vi "Network_Ping.vi"(4 "dontFragment (F)":bool, 6 "Bytes number (32)":u16=32, 8 "error in (no error)":errorcluster, 9 "Tentatives (4)":u16(ring)=4 items=["1"=1, "2"=2, "3"=3, "4"=4], 10 "TimeOut (100ms)":i32=100, 11 "Address":string="localhost") -> (0 "error out":errorcluster, 1 "Success":bool, 2 "Status":i32(ring) items=["Success"=0, "DestinationNetworkUnreachable"=11002, "DestinationHostUnreachable"=11003, "DestinationProhibited, DestinationProtocolUnreachable"=11004, "DestinationPortUnreachable"=11005, "NoResources"=11006, "BadOption"=11007, "HardwareError"=11008, "PacketTooBig"=11009, "TimedOut"=11010, "BadRoute"=11012, "TtlExpired"=11013, "TtlReassemblyTimeExceeded"=11014, "ParameterProblem"=11015, "SourceQuench"=11016, "BadDestination"=11018, "DestinationUnreachable"=11040, "TimeExceeded"=11041, "BadHeader"=11042, "UnrecognizedNextHeader"=11043, "IcmpError"=11044, "DestinationScopeMismatch"=11045, "Unknown"=-1])   [LabVIEW 2021]
doc: "This VI sends n ping to an address.\n\n.NET Technology, works only for Windows."
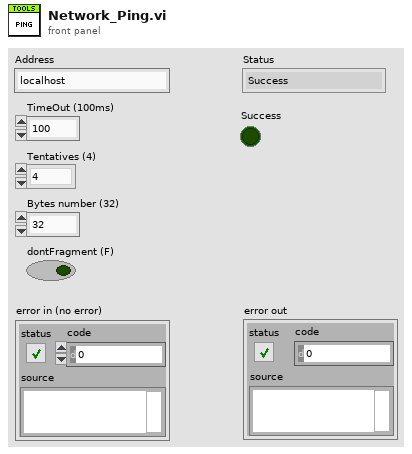
[diagram p1: front panel]
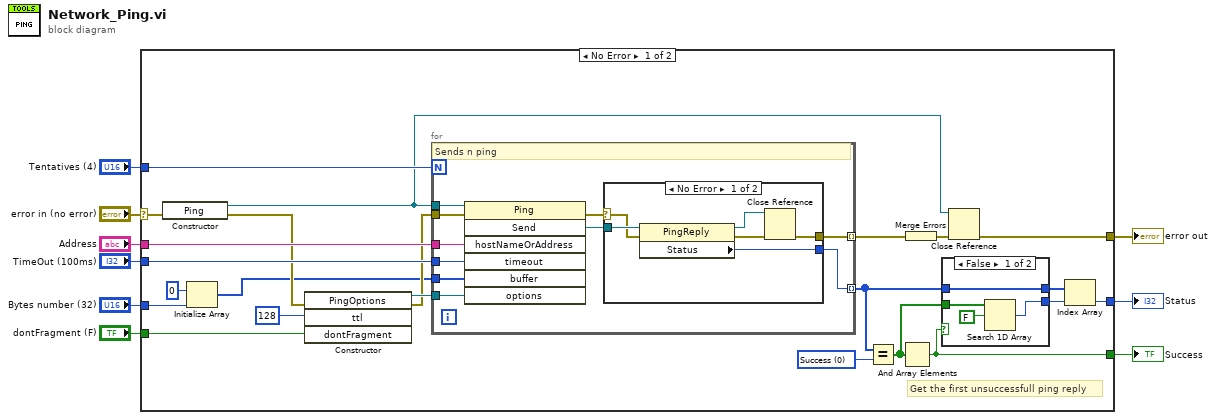
[diagram p0: block diagram]
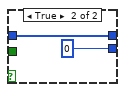
[diagram p2: hidden frame]
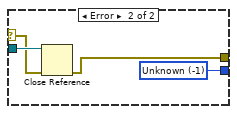
[diagram p3: hidden frame]
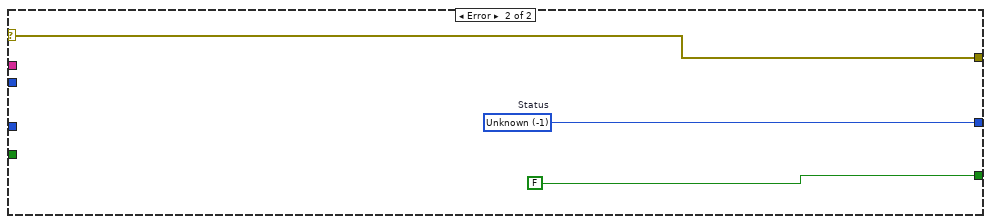
[diagram p4: hidden frame]
diagram:
  n1 = case shown="No Error" "error in (no error)" {
    selector: "error in (no error)" -> [w21 w61]
    tunnel: "Address" -> [w32 _]
    tunnel: "TimeOut (100ms)" -> [w31 _]
    tunnel: "Tentatives (4)" -> [w30 _]
    tunnel: [w26 w61] -> w6
    tunnel: [w24 FALSE] -> w5
    tunnel: [w22 w60] -> w4
    tunnel: "Bytes number (32)" -> [w14 _]
    tunnel: "dontFragment (F)" -> [w10 _]
    frame No Error {
      w19 = 0 items=["Success"=0, "DestinationNetworkUnreachable"=11002, "DestinationHostUnreachable"=11003, "DestinationProhibited, DestinationProtocolUnreachable"=11004, "DestinationPortUnreachable"=11005, "NoResources"=11006, "BadOption"=11007, "HardwareError"=11008, "PacketTooBig"=11009, "TimedOut"=11010, "BadRoute"=11012, "TtlExpired"=11013, "TtlReassemblyTimeExceeded"=11014, "ParameterProblem"=11015, "SourceQuench"=11016, "BadDestination"=11018, "DestinationUnreachable"=11040, "TimeExceeded"=11041, "BadHeader"=11042, "UnrecognizedNextHeader"=11043, "IcmpError"=11044, "DestinationScopeMismatch"=11045, "Unknown"=-1] ("Status")
      # "Get the first unsuccessfull ping reply"
      n2 = constructor class="Ping"(error in=w21) -> (reference out=w28:refnum<k24>, error out=w15:errorcluster)  [unwired: 2 in, 1 out]
      n3 = Initialize Array(u8 0, w14) -> (w12:u8[])
      n4 = constructor class="PingOptions"(error in=w15, "ttl"=128, "dontFragment"=w10) -> (reference out=w17:refnum<k24>, error out=w16:errorcluster)  [unwired: 2 in, 3 out]
      n5 = for {
        N: w30 -> [_]
        tunnel: w28 -> [w48]
        tunnel: w32 -> [w46]
        tunnel: w31 -> [w45]
        tunnel: w16 -> [w47]
        tunnel: [w42] -> w29 mode=indexing
        tunnel: [w41] -> w20 mode=indexing
        tunnel: w12 -> [w40]
        tunnel: w17 -> [w39]
        # "Sends n ping"
        n6 = invoke class="Ping" method="Send"(reference=w48, error in=w47, "hostNameOrAddress"=w46, "timeout"=w45, "buffer"=w40, "options"=w39) -> (error out=w43:errorcluster, "Send"=w44:refnum<k24>)  [unwired: 1 in, 5 out]
        n7 = case shown="No Error" w43 {
          selector: w43 -> [w53 w56]
          tunnel: w44 -> [w54 w57]
          tunnel: [w52 w58] -> w41
          tunnel: [w49 w55] -> w42
          frame No Error {
            n8 = property class="PingReply"(reference=w54, error in=w53) -> (reference out=w51:refnum<k24>, error out=w50:errorcluster, "Status"=w52:i32)
            n9 = Close Reference(reference=w51, error in (no error)=w50) -> (error out=w49:errorcluster)
          }
          frame Error {
            w58 = -1 items=["Success"=0, "DestinationNetworkUnreachable"=11002, "DestinationHostUnreachable"=11003, "DestinationProhibited, DestinationProtocolUnreachable"=11004, "DestinationPortUnreachable"=11005, "NoResources"=11006, "BadOption"=11007, "HardwareError"=11008, "PacketTooBig"=11009, "TimedOut"=11010, "BadRoute"=11012, "TtlExpired"=11013, "TtlReassemblyTimeExceeded"=11014, "ParameterProblem"=11015, "SourceQuench"=11016, "BadDestination"=11018, "DestinationUnreachable"=11040, "TimeExceeded"=11041, "BadHeader"=11042, "UnrecognizedNextHeader"=11043, "IcmpError"=11044, "DestinationScopeMismatch"=11045, "Unknown"=-1] ("Status")
            n10 = Close Reference(reference=w57, error in (no error)=w56) -> (error out=w55:errorcluster)
          }
        }
      }
      n11 = Equal?(x=w20, y=w19) -> (x = y?=w18:bool[])
      n12 = And Array Elements(Boolean array=w18) -> (logical AND=w24:bool)
      n13 = Merge Errors(w29) -> (w27:errorcluster)
      n14 = case shown="False" w24 {
        tunnel: w20 -> [w34 w38]
        tunnel: [w33 0 ("index of element")] -> w23
        tunnel: w18 -> [w35 _]
        tunnel: [w34 w38] -> w25
        frame False {
          n15 = Search 1D Array(1D array=w35, element=FALSE) -> (index of element=w33:i32)  [unwired: 1 in]
        }
        frame True {
        }
      }
      n16 = Close Reference(reference=w28, error in (no error)=w27) -> (error out=w26:errorcluster)
      n17 = Index Array(array=w25, index=w23) -> (element=w22:i32)
    }
    frame Error {
      w60 = -1 items=["Success"=0, "DestinationNetworkUnreachable"=11002, "DestinationHostUnreachable"=11003, "DestinationProhibited, DestinationProtocolUnreachable"=11004, "DestinationPortUnreachable"=11005, "NoResources"=11006, "BadOption"=11007, "HardwareError"=11008, "PacketTooBig"=11009, "TimedOut"=11010, "BadRoute"=11012, "TtlExpired"=11013, "TtlReassemblyTimeExceeded"=11014, "ParameterProblem"=11015, "SourceQuench"=11016, "BadDestination"=11018, "DestinationUnreachable"=11040, "TimeExceeded"=11041, "BadHeader"=11042, "UnrecognizedNextHeader"=11043, "IcmpError"=11044, "DestinationScopeMismatch"=11045, "Unknown"=-1]  # Status
    }
  }
  "Status" <- w4
  "Success" <- w5
  "error out" <- w6
